vi "H5_WriteAttr.vi"(0 "HDF5 Ref In":T1, 1 "X Start":sgl, 2 "X End":sgl=10.0, 3 "Y Start":sgl, 4 "Y End":sgl=8.0, 5 "Scan Mode":enum16{"Raster", "Serpentine"}(ring), 6 "Speed Control (mm/s)":sgl=1.0 min=0.1, 7 "error in (no error)":errorcluster, 8 "Scan Time (Approx.)":string, 9 "Pixel Count":i32=6 caption="X Pixels", 10 "X Step Size (R)":sgl format="%#_2g", 11 "Line Count":i32=6 caption="Y Pixels", 12 "Y Step Size (R)":sgl format="%#_2g", 13 "Gen Sampling Rate":u64, 14 "Amplitudes (V)":sgl[](array[numeric]) format="%#_2g", 16 "Offset":sgl format="%#_2g", 17 "Gain":sgl format="%#_2g", 18 "Waves per Pixel":u16, 19 "Record Size":u16=1024, 21 "Delay(us)":sgl min=0 step=0.1 format="%#_4g", 22 "Sampling Freq (Hz)":sgl min=0 step=0.1 format="%#_4g", 23 "Temperature":sgl min=0 step=0.1 format="%#_4g", 24 "Remarks":string="Notes: Scanned in UiT", 25 "Transducer Freq(Hz)":u64 step=1, 26 "Immersion Medium":string="Water") -> (20 "HDF5 Ref Out":T1, 27 "error out":errorcluster)   [LabVIEW 2020]
uses:
  <vilib>/UPVI/lvhdf5/library.llb/HDF5 Ref.ctl
  <vilib>/UPVI/lvhdf5/group.llb/OpenCreateGroup (String).vi
  <vilib>/UPVI/lvhdf5/attribute.llb/Write Multiple Attributes.vi
  <vilib>/UPVI/lvhdf5/attribute.llb/LVH5A Operation.ctl
  <vilib>/UPVI/lvhdf5/attribute.llb/LVH5 Write Attributes.xnode
  <vilib>/Utility/VariantDataType/GetClusterInfo.vi
  <vilib>/Utility/VariantDataType/VariantType.lvlib
  <vilib>/Utility/VariantDataType/GetTypeInfo.vi
  <vilib>/UPVI/lvhdf5/attribute.llb/Cluster to Attribute Array.xnode
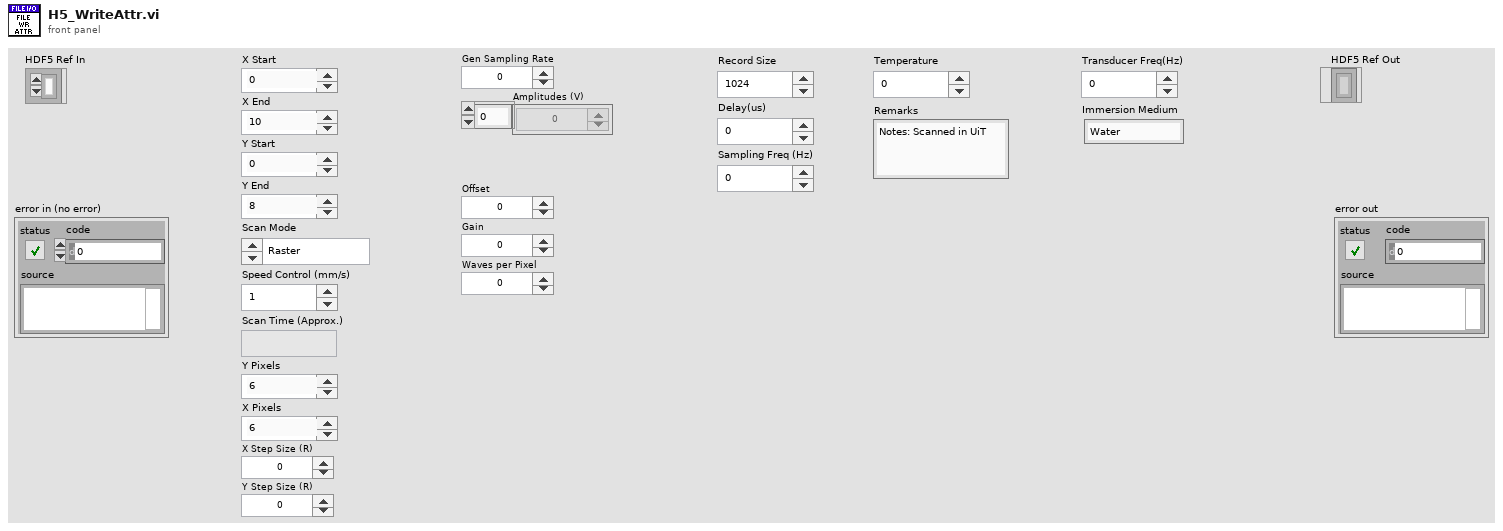
[diagram p1: front panel]
types:
  T1 = typedef "HDF5 Ref.ctl" = refnum<k1>
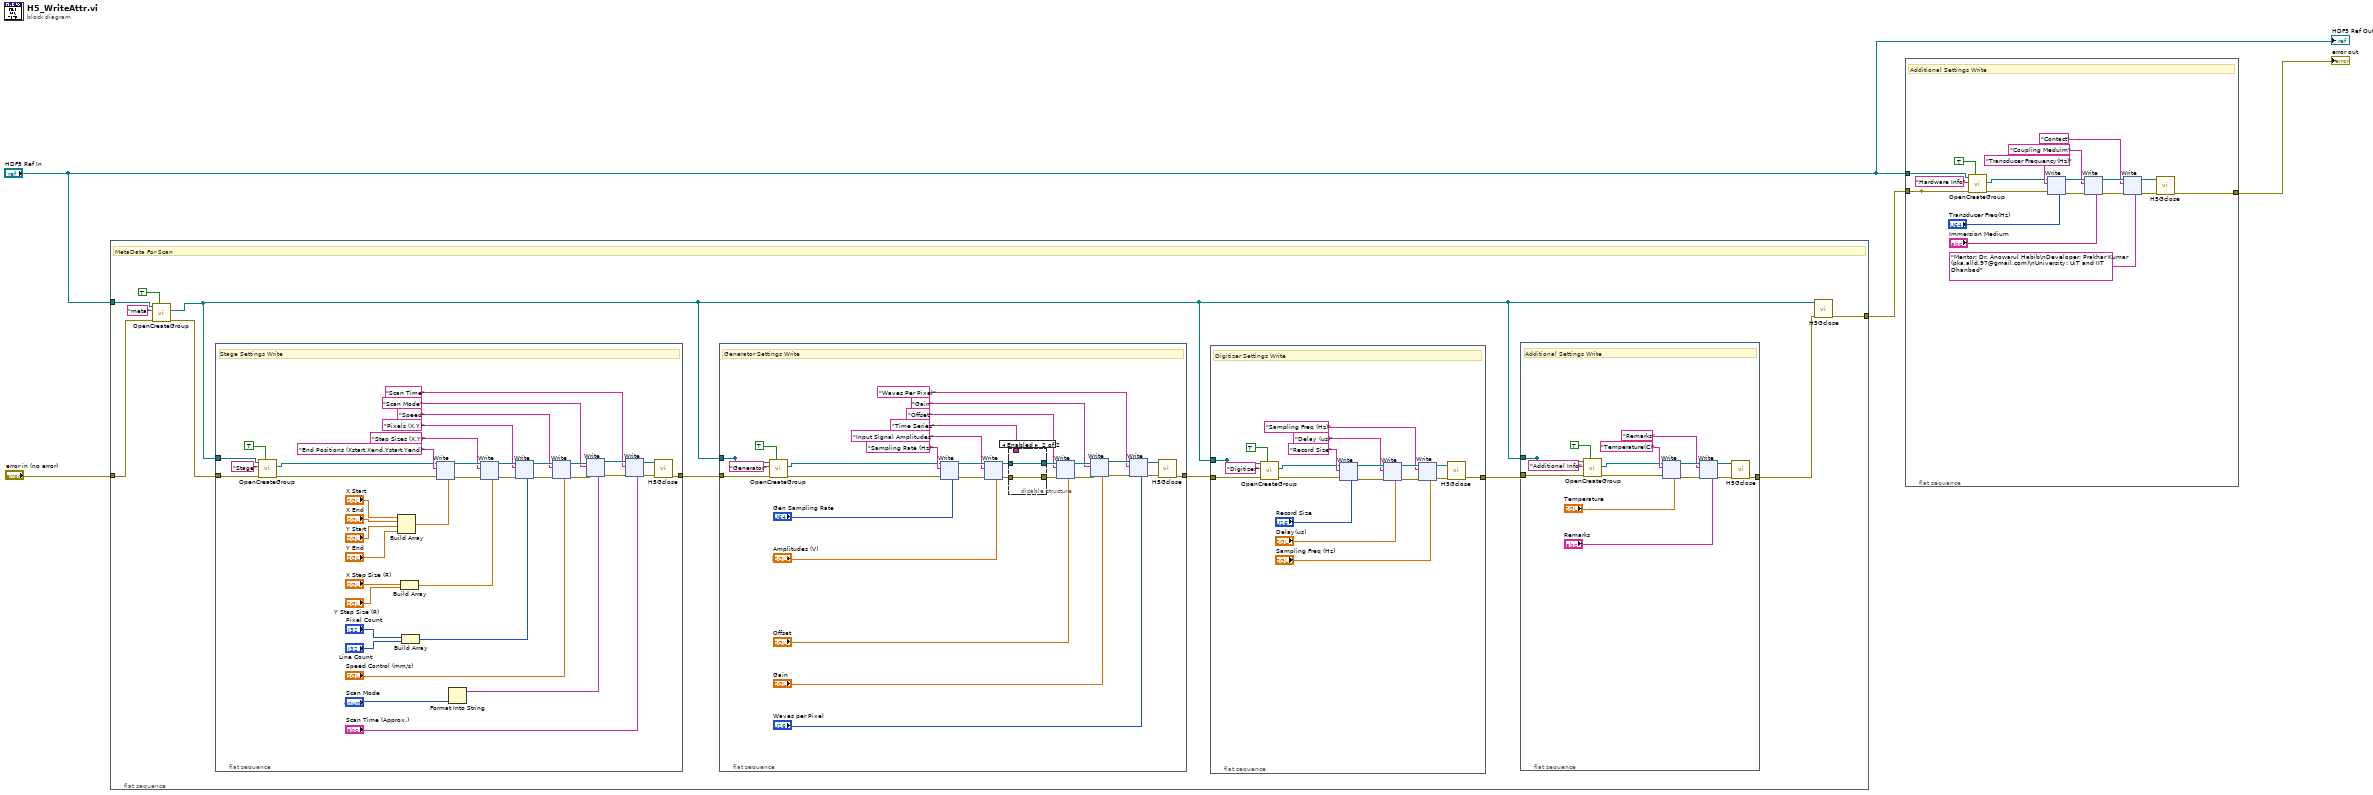
[diagram p0: block diagram]
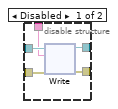
[diagram p2: hidden frame]
diagram:
  n1 = flat-sequence {
    tunnel: "error in (no error)" -> [w10]
    tunnel: "HDF5 Ref In" -> [w12]
    tunnel: [w6] -> w3
    frame #0 {
      # "MetaData For Scan"
      n2 = call-poly <vilib>:"OpenCreateGroup.vi"("Create if not found (F)"=TRUE, "error in (no error)"=w10, "Group"="meta", "HDF5 Ref"=w12) -> ("error out"=w11:errorcluster, "HDF5 Group Ref"=w8:T1)  [unwired: 5 in, 1 out]
      n3 = flat-sequence {
        tunnel: w11 -> [w1345]
        tunnel: w8 -> [w1344]
        tunnel: [w1342] -> w15
        frame #0 {
          # "Stage Settings Write"
          n4 = call-poly <vilib>:"OpenCreateGroup.vi"("Create if not found (F)"=TRUE, "error in (no error)"=w1345, "Group"="Stage", "HDF5 Ref"=w1344) -> ("error out"=w1349:errorcluster, "HDF5 Group Ref"=w1348:T1)  [unwired: 5 in, 1 out]
          n5 = Build Array("X Start", "X End", "Y Start", "Y End") -> (w1371:sgl[])
          n6 = Build Array("X Step Size (R)", "Y Step Size (R)") -> (w1359:sgl[])
          n7 = Build Array("Pixel Count", "Line Count") -> (w1358:i32[])
          n8 = xnode "Write"("HDF5 Ref"=w1348, "error in (no error)"=w1349, "Name(s)"="End Positions (Xstart,Xend,Ystart,Yend)", "Value(s)"=w1371) -> ("HDF5 Ref out"=w1370:T1, "error out"=w1369:errorcluster)  [unwired: 1 in]
          n9 = Format Into String("Scan Mode") -> (resulting string=w1351:string)  [unwired: 3 in, 1 out]
          n10 = xnode "Write"("HDF5 Ref"=w1370, "error in (no error)"=w1369, "Name(s)"="Step Sizes (X,Y)", "Value(s)"=w1359) -> ("HDF5 Ref out"=w1368:T1, "error out"=w1367:errorcluster)  [unwired: 1 in]
          n11 = xnode "Write"("HDF5 Ref"=w1368, "error in (no error)"=w1367, "Name(s)"="Pixels (X,Y)", "Value(s)"=w1358) -> ("HDF5 Ref out"=w1366:T1, "error out"=w1365:errorcluster)  [unwired: 1 in]
          n12 = xnode "Write"("HDF5 Ref"=w1366, "error in (no error)"=w1365, "Name(s)"="Speed", "Value(s)"="Speed Control (mm/s)") -> ("HDF5 Ref out"=w1364:T1, "error out"=w1363:errorcluster)  [unwired: 1 in]
          n13 = xnode "Write"("HDF5 Ref"=w1364, "error in (no error)"=w1363, "Name(s)"="Scan Mode", "Value(s)"=w1351) -> ("HDF5 Ref out"=w1362:T1, "error out"=w1361:errorcluster)  [unwired: 1 in]
          n14 = xnode "Write"("HDF5 Ref"=w1362, "error in (no error)"=w1361, "Name(s)"="Scan Time", "Value(s)"="Scan Time (Approx.)") -> ("HDF5 Ref out"=w1341:T1, "error out"=w1343:errorcluster)  [unwired: 1 in]
          n15 = call <vilib>:"H5Gclose.vi"("error in (no error)"=w1343, "HDF5 Group Ref"=w1341) -> ("error out"=w1342:errorcluster)  [unwired: 7 in]
        }
      }
      n16 = flat-sequence {
        tunnel: w15 -> [w629]
        tunnel: [w625] -> _
        tunnel: [w627] -> w14
        tunnel: w8 -> [w625]
        frame #0 {
          # "Generator Settings Write"
          n17 = call-poly <vilib>:"OpenCreateGroup.vi"("Create if not found (F)"=TRUE, "error in (no error)"=w629, "Group"="Generator", "HDF5 Ref"=w625) -> ("error out"=w633:errorcluster, "HDF5 Group Ref"=w632:T1)  [unwired: 5 in, 1 out]
          n18 = xnode "Write"("HDF5 Ref"=w632, "error in (no error)"=w633, "Name(s)"="Sampling Rate (Hz)", "Value(s)"="Gen Sampling Rate") -> ("HDF5 Ref out"=w648:T1, "error out"=w647:errorcluster)  [unwired: 1 in]
          n19 = xnode "Write"("HDF5 Ref"=w648, "error in (no error)"=w647, "Name(s)"="Input Signal Amplitudes", "Value(s)"="Amplitudes (V)") -> ("HDF5 Ref out"=w646:T1, "error out"=w645:errorcluster)  [unwired: 1 in]
          n20 = disable-structure shown="Enabled" {
            disable-tunnel: w646 -> [w654 w770]
            disable-tunnel: w645 -> [w653 w769]
            disable-tunnel: [w652 w770] -> w644
            disable-tunnel: [w651 w769] -> w643
            disable-tunnel: "Time Series" -> [w650 _]
            frame Disabled {
              n21 = xnode "Write"("HDF5 Ref"=w654, "error in (no error)"=w653, "Name(s)"=w650) -> ("HDF5 Ref out"=w652:T1, "error out"=w651:errorcluster)  [unwired: 2 in]
            }
            frame Enabled {
            }
          }
          n22 = xnode "Write"("HDF5 Ref"=w644, "error in (no error)"=w643, "Name(s)"="Offset", "Value(s)"="Offset") -> ("HDF5 Ref out"=w642:T1, "error out"=w641:errorcluster)  [unwired: 1 in]
          n23 = xnode "Write"("HDF5 Ref"=w642, "error in (no error)"=w641, "Name(s)"="Gain", "Value(s)"="Gain") -> ("HDF5 Ref out"=w640:T1, "error out"=w639:errorcluster)  [unwired: 1 in]
          n24 = xnode "Write"("HDF5 Ref"=w640, "error in (no error)"=w639, "Name(s)"="Waves Per Pixel", "Value(s)"="Waves per Pixel") -> ("HDF5 Ref out"=w626:T1, "error out"=w628:errorcluster)  [unwired: 1 in]
          n25 = call <vilib>:"H5Gclose.vi"("error in (no error)"=w628, "HDF5 Group Ref"=w626) -> ("error out"=w627:errorcluster)  [unwired: 7 in]
        }
      }
      n26 = flat-sequence {
        tunnel: w14 -> [w264]
        tunnel: w8 -> [w262]
        tunnel: [w263] -> w9
        tunnel: [w262] -> _
        frame #0 {
          # "Digitizer Settings Write"
          n27 = call-poly <vilib>:"OpenCreateGroup.vi"("Create if not found (F)"=TRUE, "error in (no error)"=w264, "Group"="Digitizer", "HDF5 Ref"=w262) -> ("error out"=w268:errorcluster, "HDF5 Group Ref"=w267:T1)  [unwired: 5 in, 1 out]
          n28 = xnode "Write"("HDF5 Ref"=w267, "error in (no error)"=w268, "Name(s)"="Record Size", "Value(s)"="Record Size") -> ("HDF5 Ref out"=w276:T1, "error out"=w275:errorcluster)  [unwired: 1 in]
          n29 = xnode "Write"("HDF5 Ref"=w276, "error in (no error)"=w275, "Name(s)"="Delay (us)", "Value(s)"="Delay(us)") -> ("HDF5 Ref out"=w274:T1, "error out"=w273:errorcluster)  [unwired: 1 in]
          n30 = xnode "Write"("HDF5 Ref"=w274, "error in (no error)"=w273, "Name(s)"="Sampling Freq (Hz)", "Value(s)"="Sampling Freq (Hz)") -> ("HDF5 Ref out"=w272:T1, "error out"=w271:errorcluster)  [unwired: 1 in]
          n31 = call <vilib>:"H5Gclose.vi"("error in (no error)"=w271, "HDF5 Group Ref"=w272) -> ("error out"=w263:errorcluster)  [unwired: 7 in]
        }
      }
      n32 = flat-sequence {
        tunnel: w9 -> [w20]
        tunnel: w8 -> [w18]
        tunnel: [w19] -> w7
        tunnel: [w18] -> _
        frame #0 {
          # "Additional Settings Write"
          n33 = call-poly <vilib>:"OpenCreateGroup.vi"("Create if not found (F)"=TRUE, "error in (no error)"=w20, "Group"="Additional Info", "HDF5 Ref"=w18) -> ("error out"=w24:errorcluster, "HDF5 Group Ref"=w23:T1)  [unwired: 5 in, 1 out]
          n34 = xnode "Write"("HDF5 Ref"=w23, "error in (no error)"=w24, "Name(s)"="Temperature(C)", "Value(s)"="Temperature") -> ("HDF5 Ref out"=w29:T1, "error out"=w28:errorcluster)  [unwired: 1 in]
          n35 = xnode "Write"("HDF5 Ref"=w29, "error in (no error)"=w28, "Name(s)"="Remarks", "Value(s)"="Remarks") -> ("HDF5 Ref out"=w27:T1, "error out"=w26:errorcluster)  [unwired: 1 in]
          n36 = call <vilib>:"H5Gclose.vi"("error in (no error)"=w26, "HDF5 Group Ref"=w27) -> ("error out"=w19:errorcluster)  [unwired: 7 in]
        }
      }
      n37 = call <vilib>:"H5Gclose.vi"("error in (no error)"=w7, "HDF5 Group Ref"=w8) -> ("error out"=w6:errorcluster)  [unwired: 7 in]
    }
  }
  n38 = flat-sequence {
    tunnel: [w2071] -> _
    tunnel: [w2075] -> w1
    tunnel: "HDF5 Ref In" -> [w2074]
    tunnel: w3 -> [w2071]
    frame #0 {
      # "Additional Settings Write"
      n39 = call-poly <vilib>:"OpenCreateGroup.vi"("Create if not found (F)"=TRUE, "error in (no error)"=w2071, "Group"="Hardware Info", "HDF5 Ref"=w2074) -> ("error out"=w2079:errorcluster, "HDF5 Group Ref"=w2078:T1)  [unwired: 5 in, 1 out]
      n40 = xnode "Write"("HDF5 Ref"=w2078, "error in (no error)"=w2079, "Name(s)"="Transducer Frequency(Hz)", "Value(s)"="Transducer Freq(Hz)") -> ("HDF5 Ref out"=w2082:T1, "error out"=w2081:errorcluster)  [unwired: 1 in]
      n41 = xnode "Write"("HDF5 Ref"=w2082, "error in (no error)"=w2081, "Name(s)"="Coupling Meduim", "Value(s)"="Immersion Medium") -> ("HDF5 Ref out"=w2070:T1, "error out"=w2069:errorcluster)  [unwired: 1 in]
      n42 = xnode "Write"("HDF5 Ref"=w2070, "error in (no error)"=w2069, "Name(s)"="Contact", "Value(s)"="Mentor: Dr. Anowarul Habib\nDeveloper: Prakhar Kumar (pka.alld.97@gmail.com)\nUniversity: UiT and IIT Dhanbad" ("Group")) -> ("HDF5 Ref out"=w2068:T1, "error out"=w2067:errorcluster)  [unwired: 1 in]
      n43 = call <vilib>:"H5Gclose.vi"("error in (no error)"=w2067, "HDF5 Group Ref"=w2068) -> ("error out"=w2075:errorcluster)  [unwired: 7 in]
    }
  }
  "error out" <- w1
  "HDF5 Ref Out" <- "HDF5 Ref In"
